vi "Compass.vi"() -> ()   [LabVIEW 2009]
uses:
  <vilib>/Instr/_visa.llb/VISA Configure Serial Port (Instr).vi
panel:
  out "Compass Period (ms)":u16
  in  "Compass Tick Count(mSec)":u16
  out "Compass error out":errorcluster
  out "pitch buffer":u8[](array[numeric])
  out "heading data":u8[](array[numeric])
  out "heading buffer":u8[](array[numeric])
  out "roll data":u8[](array[numeric])
  out "roll buffer":u8[](array[numeric])
  out "pitch data":u8[](array[numeric])
  out "Compass read count":i32
  out "Compass comma count":i32
  out "Compass Heartbeat":bool
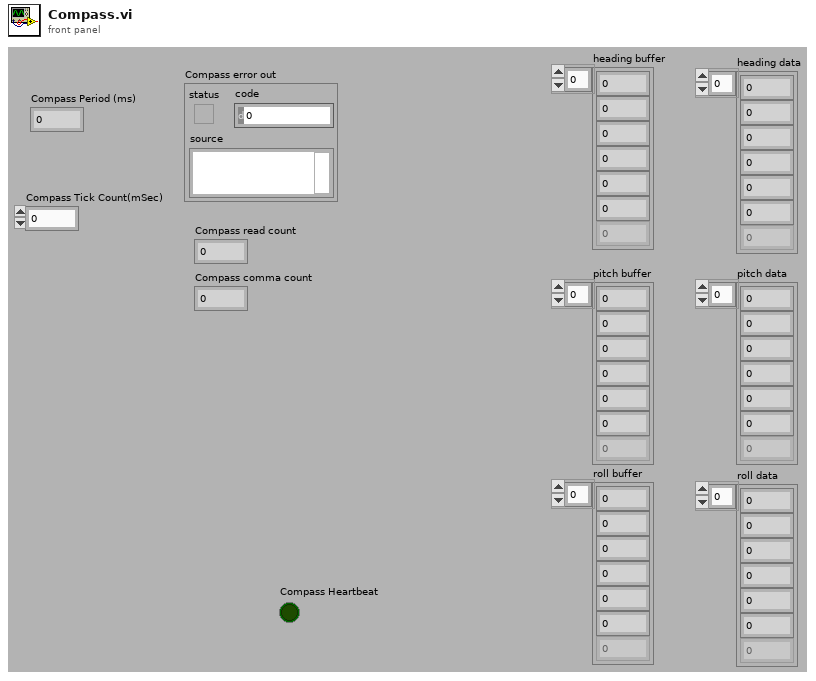
[diagram p1: front panel]
types:
  T1 = enum16{"Search for LF", "Read heading", "Read pitch", "Read roll"}
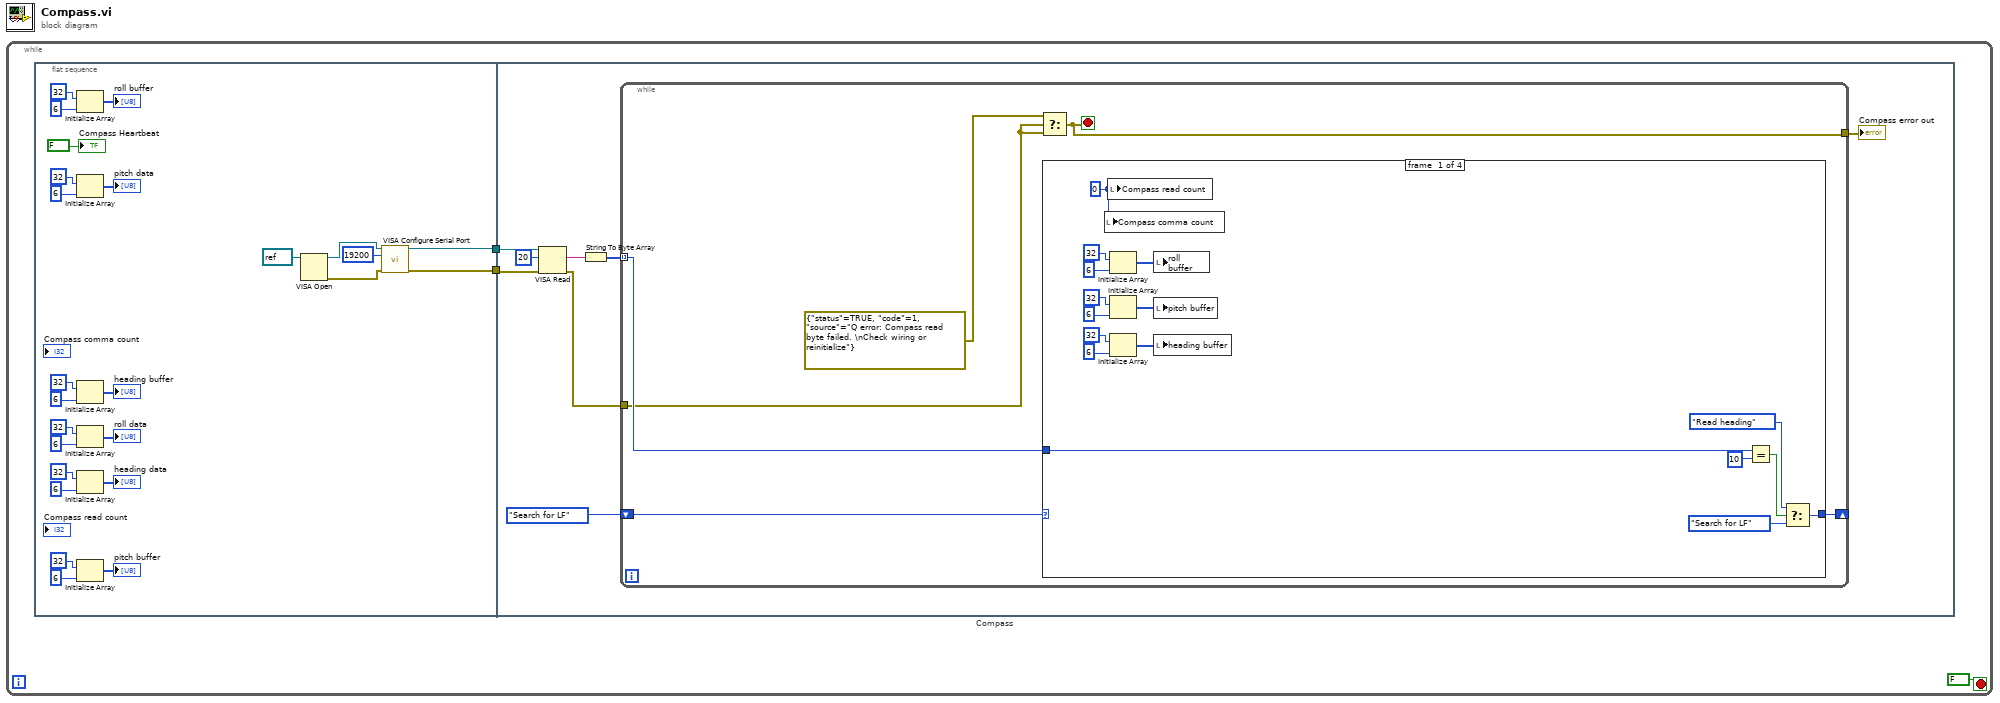
[diagram p0: block diagram]
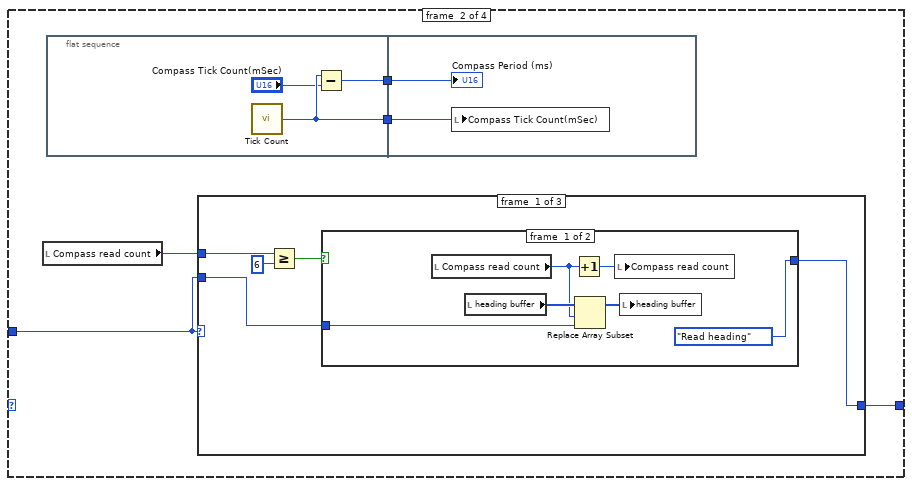
[diagram p2: hidden frame]
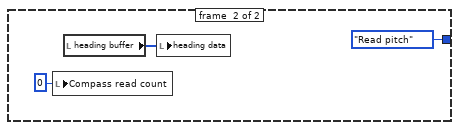
[diagram p3: hidden frame]
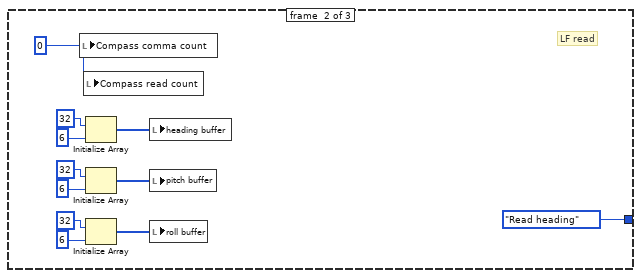
[diagram p4: hidden frame]
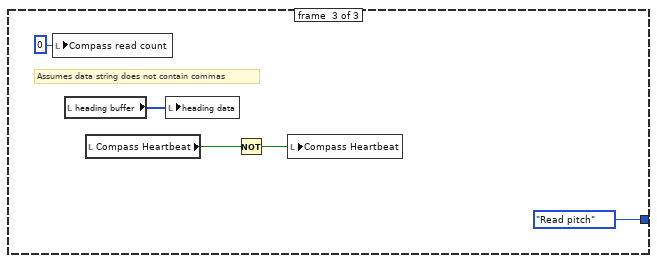
[diagram p5: hidden frame]
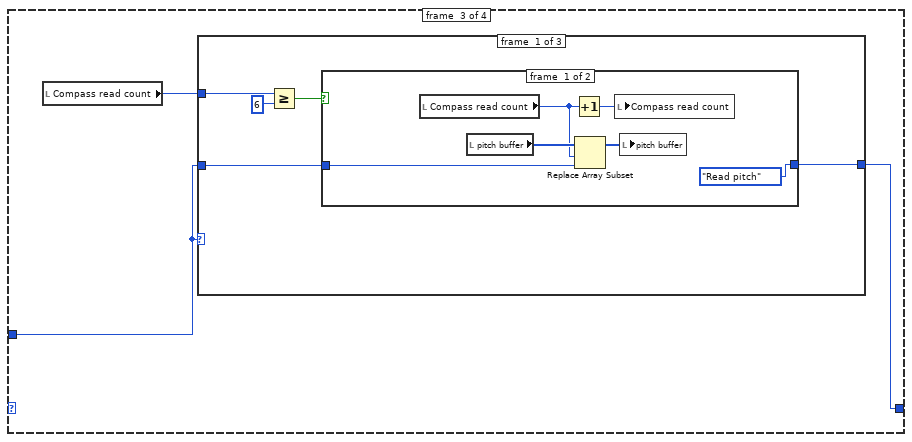
[diagram p6: hidden frame]
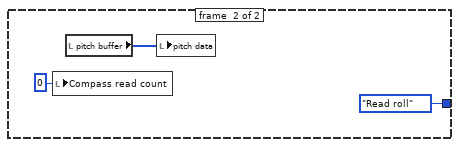
[diagram p7: hidden frame]
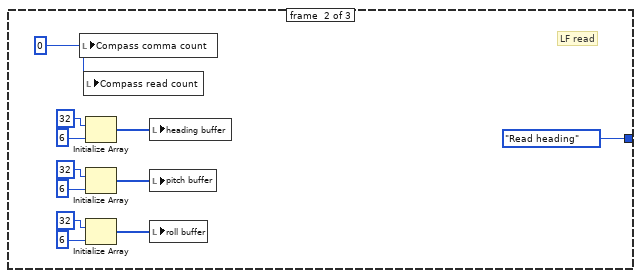
[diagram p8: hidden frame]
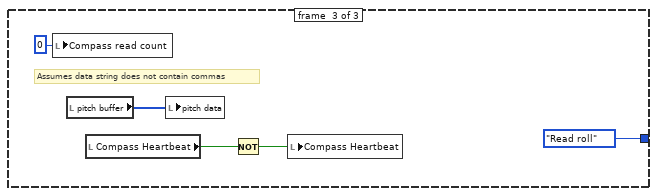
[diagram p9: hidden frame]
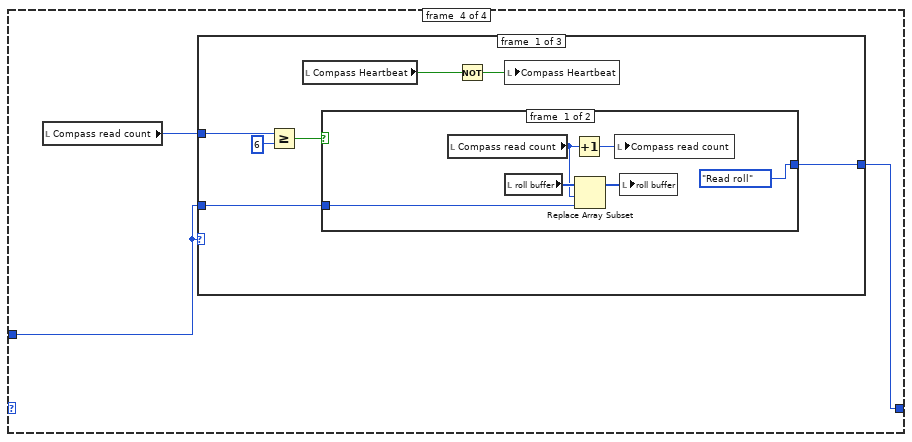
[diagram p10: hidden frame]
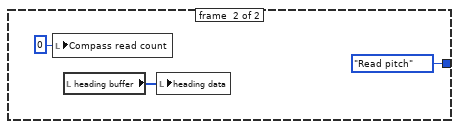
[diagram p11: hidden frame]
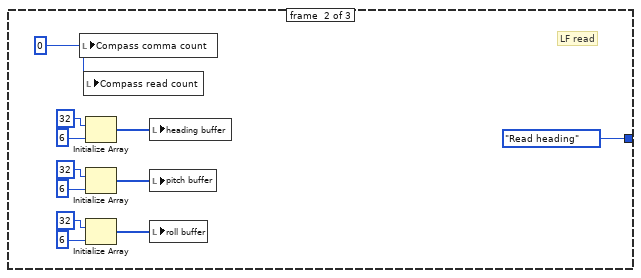
[diagram p12: hidden frame]
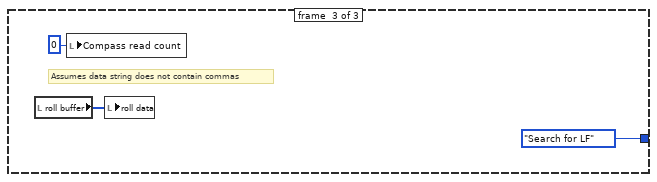
[diagram p13: hidden frame]
diagram:
  n1 = while {
    stop <- FALSE stop-if-true
    n2 = flat-sequence "Compass" {
      tunnel: [w5] -> w3
      tunnel: [w4] -> w1
      tunnel: w3 -> [w34]
      tunnel: w1 -> [w33]
      frame #0 {
        n3 = Initialize Array(u8 32 ("y"), 6 ("dimension size")) -> (→"roll buffer":u8[])
        n4 = Initialize Array(u8 32 ("y"), 6 ("dimension size")) -> (→"pitch data":u8[])
        n5 = Initialize Array(u8 32 ("y"), 6 ("dimension size")) -> (→"heading buffer":u8[])
        n6 = Initialize Array(u8 32 ("y"), 6 ("dimension size")) -> (→"roll data":u8[])
        n7 = Initialize Array(u8 32 ("y"), 6 ("dimension size")) -> (→"heading data":u8[])
        n8 = Initialize Array(u8 32 ("y"), 6 ("dimension size")) -> (→"pitch buffer":u8[])
        n9 = VISA Open(VISA resource name=refnum<visa-resource-name> refnum) -> (VISA resource name=w7:refnum<visa-resource-name>, error out=w6:errorcluster)  [unwired: 4 in]
        n10 = call-poly "VISA Configure Serial Port"("VISA resource name"=w7, "baud rate (9600)"=u32 19200, "error in (no error)"=w6) -> ("VISA resource name out"=w5:refnum<visa-resource-name>, "error out"=w4:errorcluster)  [unwired: 11 in]
        "Compass Heartbeat" <- FALSE ("SICK Heartbeat")
      }
      frame #1 {
        n11 = VISA Read(VISA resource name=w34, byte count=u32 20, error in (no error)=w33) -> (read buffer=w31:string, error out=w29:errorcluster)  [unwired: 2 out]
        n12 = String To Byte Array(string=w31) -> (unsigned byte array=w30:u8[])
        n13 = while {
          shift-right: [w41] -> _
          shift-left: T1."Search for LF" ("Main states") -> [w42]
          tunnel: [w39] -> w36
          tunnel: w30 -> [w38] mode=indexing
          tunnel: w29 -> [w37]
          stop <- w39 stop-if-true
          n14 = Select(t=errorcluster {"status"=TRUE, "code"=1, "source"="Q error: Compass read byte failed. \nCheck wiring or reinitialize"} ("error out"), s=w37, f=w37) -> (s? t:f=w39:errorcluster)
          n15 = case shown="\"Search for LF\", Default" w42 {
            tunnel: w38 -> [w58 w62 w100 w133]
            tunnel: [w55 w63 w101 w134] -> w41
            frame #0 {
              w50 = 0
              n16 = local write "Compass comma count"(w50) -> ()
              n17 = local write "Compass read count"(w50) -> ()
              n18 = Initialize Array(u8 32 ("y"), 6 ("dimension size")) -> (w45:u8[])
              n19 = Initialize Array(u8 32 ("y"), 6 ("dimension size")) -> (w44:u8[])
              n20 = Initialize Array(u8 32 ("y"), 6 ("dimension size")) -> (w43:u8[])
              n21 = local write "roll buffer"(w45) -> ()
              n22 = local write "pitch buffer"(w44) -> ()
              n23 = local write "heading buffer"(w43) -> ()
              n24 = Equal?(x=w58, y=u8 10) -> (x = y?=w56:bool)
              n25 = Select(t=T1."Read heading" ("Main states"), s=w56, f=T1."Search for LF" ("Main states")) -> (s? t:f=w55:T1)
            }
            frame #1 {
              n26 = local read "Compass read count"() -> (w61:i32)
              n27 = flat-sequence {
                tunnel: [w66] -> w60
                tunnel: [w64] -> w59
                tunnel: w60 -> [w68]
                tunnel: w59 -> [w67]
                frame #0 {
                  n28 = call "Tick Count"() -> ("Tick Count(mSec)"=w66:u16)
                  n29 = Subtract(x=w66, y="Compass Tick Count(mSec)") -> (x-y=w64:u16)
                }
                frame #1 {
                  n30 = local write "Compass Tick Count(mSec)"(w68) -> ()
                  "Compass Period (ms)" <- w67
                }
              }
              n31 = case shown="0, Default" w62 {
                tunnel: [w72 T1."Read heading" ("Main states") T1."Read pitch" ("Main states")] -> w63
                tunnel: w62 -> [w73 _ _]
                tunnel: w61 -> [w71 _ _]
                frame #0 {
                  n32 = Greater Or Equal?(x=w71, y=6) -> (x >= y?=w69:bool)
                  n33 = case shown="False" w69 {
                    tunnel: w73 -> [w75 _]
                    tunnel: [T1."Read heading" ("Main states") T1."Read pitch" ("Main states")] -> w72
                    frame #0 {
                      n34 = local read "Compass read count"() -> (w77:i32)
                      n35 = local read "heading buffer"() -> (w78:u8[])
                      n36 = Increment(x=w77) -> (x+1=w79:i32)
                      n37 = Replace Array Subset(array=w78, new element=w75, index=w77) -> (w76:u8[])
                      n38 = local write "Compass read count"(w79) -> ()
                      n39 = local write "heading buffer"(w76) -> ()
                    }
                    frame #1 {
                      n40 = local write "Compass read count"(0 ("Read count")) -> ()
                      n41 = local read "heading buffer"() -> (w82:u8[])
                      n42 = local write "heading data"(w82) -> ()
                    }
                  }
                }
                frame #1 {
                  w90 = 0 ("Comma count")
                  # "LF read"
                  n43 = local write "Compass comma count"(w90) -> ()
                  n44 = local write "Compass read count"(w90) -> ()
                  n45 = Initialize Array(u8 32 ("y"), 6 ("dimension size")) -> (w91:u8[])
                  n46 = Initialize Array(u8 32 ("y"), 6 ("dimension size")) -> (w85:u8[])
                  n47 = Initialize Array(u8 32 ("y"), 6 ("dimension size")) -> (w84:u8[])
                  n48 = local write "heading buffer"(w91) -> ()
                  n49 = local write "pitch buffer"(w85) -> ()
                  n50 = local write "roll buffer"(w84) -> ()
                }
                frame #2 {
                  # "Assumes data string does not contain commas"
                  n51 = local write "Compass read count"(0 ("Comma count")) -> ()
                  n52 = local read "heading buffer"() -> (w98:u8[])
                  n53 = local read "Compass Heartbeat"() -> (w95:bool)
                  n54 = local write "heading data"(w98) -> ()
                  n55 = Not(x=w95) -> (.not. x?=w94:bool)
                  n56 = local write "Compass Heartbeat"(w94) -> ()
                }
              }
            }
            frame #2 {
              n57 = local read "Compass read count"() -> (w99:i32)
              n58 = case shown="44" w100 {
                tunnel: [w105 T1."Read heading" ("Main states") T1."Read roll" ("Main states")] -> w101
                tunnel: w100 -> [w106 _ _]
                tunnel: w99 -> [w104 _ _]
                frame #0 {
                  n59 = Greater Or Equal?(x=w104, y=6) -> (x >= y?=w102:bool)
                  n60 = case shown="True" w102 {
                    tunnel: w106 -> [w108 _]
                    tunnel: [T1."Read pitch" ("Main states") T1."Read roll" ("Main states")] -> w105
                    frame #0 {
                      n61 = local read "Compass read count"() -> (w110:i32)
                      n62 = local read "pitch buffer"() -> (w111:u8[])
                      n63 = Increment(x=w110) -> (x+1=w112:i32)
                      n64 = Replace Array Subset(array=w111, new element=w108, index=w110) -> (w109:u8[])
                      n65 = local write "Compass read count"(w112) -> ()
                      n66 = local write "pitch buffer"(w109) -> ()
                    }
                    frame #1 {
                      n67 = local write "Compass read count"(0 ("Read count")) -> ()
                      n68 = local read "pitch buffer"() -> (w115:u8[])
                      n69 = local write "pitch data"(w115) -> ()
                    }
                  }
                }
                frame #1 {
                  w123 = 0 ("Comma count")
                  # "LF read"
                  n70 = local write "Compass comma count"(w123) -> ()
                  n71 = local write "Compass read count"(w123) -> ()
                  n72 = Initialize Array(u8 32 ("y"), 6 ("dimension size")) -> (w124:u8[])
                  n73 = Initialize Array(u8 32 ("y"), 6 ("dimension size")) -> (w118:u8[])
                  n74 = Initialize Array(u8 32 ("y"), 6 ("dimension size")) -> (w117:u8[])
                  n75 = local write "heading buffer"(w124) -> ()
                  n76 = local write "pitch buffer"(w118) -> ()
                  n77 = local write "roll buffer"(w117) -> ()
                }
                frame #2 {
                  # "Assumes data string does not contain commas"
                  n78 = local write "Compass read count"(0 ("Comma count")) -> ()
                  n79 = local read "pitch buffer"() -> (w131:u8[])
                  n80 = local read "Compass Heartbeat"() -> (w128:bool)
                  n81 = local write "pitch data"(w131) -> ()
                  n82 = Not(x=w128) -> (.not. x?=w127:bool)
                  n83 = local write "Compass Heartbeat"(w127) -> ()
                }
              }
            }
            frame #3 {
              n84 = local read "Compass read count"() -> (w132:i32)
              n85 = case shown="0, Default" w133 {
                tunnel: [w140 T1."Read heading" ("Main states") T1."Search for LF" ("Main states")] -> w134
                tunnel: w133 -> [w141 _ _]
                tunnel: w132 -> [w139 _ _]
                frame #0 {
                  n86 = Greater Or Equal?(x=w139, y=6) -> (x >= y?=w137:bool)
                  n87 = local read "Compass Heartbeat"() -> (w136:bool)
                  n88 = case shown="False" w137 {
                    tunnel: w141 -> [w143 _]
                    tunnel: [T1."Read roll" ("Main states") T1."Read pitch" ("Main states")] -> w140
                    frame #0 {
                      n89 = local read "Compass read count"() -> (w145:i32)
                      n90 = local read "roll buffer"() -> (w146:u8[])
                      n91 = Increment(x=w145) -> (x+1=w147:i32)
                      n92 = Replace Array Subset(array=w146, new element=w143, index=w145) -> (w144:u8[])
                      n93 = local write "Compass read count"(w147) -> ()
                      n94 = local write "roll buffer"(w144) -> ()
                    }
                    frame #1 {
                      n95 = local write "Compass read count"(0 ("Read count")) -> ()
                      n96 = local read "heading buffer"() -> (w150:u8[])
                      n97 = local write "heading data"(w150) -> ()
                    }
                  }
                  n98 = Not(x=w136) -> (.not. x?=w135:bool)
                  n99 = local write "Compass Heartbeat"(w135) -> ()
                }
                frame #1 {
                  w158 = 0 ("Comma count")
                  # "LF read"
                  n100 = local write "Compass comma count"(w158) -> ()
                  n101 = local write "Compass read count"(w158) -> ()
                  n102 = Initialize Array(u8 32 ("y"), 6 ("dimension size")) -> (w159:u8[])
                  n103 = Initialize Array(u8 32 ("y"), 6 ("dimension size")) -> (w153:u8[])
                  n104 = Initialize Array(u8 32 ("y"), 6 ("dimension size")) -> (w152:u8[])
                  n105 = local write "heading buffer"(w159) -> ()
                  n106 = local write "pitch buffer"(w153) -> ()
                  n107 = local write "roll buffer"(w152) -> ()
                }
                frame #2 {
                  # "Assumes data string does not contain commas"
                  n108 = local read "roll buffer"() -> (w164:u8[])
                  n109 = local write "Compass read count"(0 ("Comma count")) -> ()
                  n110 = local write "roll data"(w164) -> ()
                }
              }
            }
          }
        }
        "Compass error out" <- w36
      }
    }
  }
